vi "DATA路径.vi"(10 "文件名":string) -> (2 "DATA路径":path)   [LabVIEW 2014]
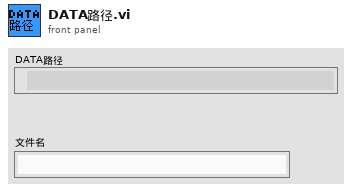
[diagram p1: front panel]
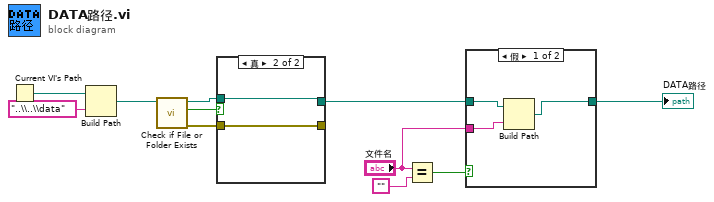
[diagram p0: block diagram]
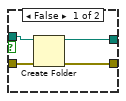
[diagram p3: hidden frame]
diagram:
  n1 = Current VI's Path() -> (path=w11:path)
  n2 = Build Path(base path=w11, name or relative path="..\\..\\data" ("名称或相对路径")) -> (appended path=w9:path)
  n3 = call <vilib>:"Check if File or Folder Exists.vi"("path"=w9) -> ("error out"=w6:errorcluster, "file or folder exists?"=w8:bool, "dup path"=w7:path)  [unwired: 8 in]
  n4 = case shown="真" w8 {
    tunnel: w7 -> [w15 w17]
    tunnel: w6 -> [w14 w16]
    tunnel: [w13 w16] -> _
    tunnel: [w12 w17] -> w3
    frame False {
      n5 = Create Folder(path (use dialog)=w15, error in=w14) -> (created path=w12:path, error out=w13:errorcluster)  [unwired: 1 in, 1 out]
    }
    frame True {
    }
  }
  n6 = Equal?(x="文件名", y="") -> (x = y?=w4:bool)
  n7 = case shown="假" w4 {
    tunnel: w3 -> [w20 w21]
    tunnel: [w18 w21] -> w2
    tunnel: "文件名" -> [w19 _]
    frame False {
      n8 = Build Path(base path=w20, name or relative path=w19) -> (appended path=w18:path)
    }
    frame True {
    }
  }
  "DATA路径" <- w2
